vi "SetTimestampFormat.vi"(6 "time column mode (0: Empty)":T1, 8 "error in (no error)":errorcluster, 9 "absolulte time (T)":bool=TRUE, 10 "timestamp format":string, 11 "Excel refnum":T2) -> (0 "error out":errorcluster, 3 "Excel refnum out":T2)   [LabVIEW 2017, in "NI_ExcelFile.lvlib"]
doc: "Sets the time column mode and the format for every time column ( not written by the user) in a .xlsx file. Time column is used to record the time when writing data.\n \n\nExcel refnum: Specifies a reference to the .xlsx file on which to perform the operation. Use the Create VI to create or open the refnum.\n\ntimestamp format: Specifies the format for the time column. For example: YYYY/MM/DD hh:mm:ss.\n\nabsolute time: Specifies whether you want to use absolute or relative time for the data in the .xlsx file. If the value is TRUE, the time in the .xlsx file starts from the current time. If the value is FALSE, the time starts from 1904/01/01 00:00:00. The default is TRUE.This control is not valid if the data type is DDT or waveform because these data types already contain time information. \n\ntime column mode: Specifies whether you want to add time columns to the .xlsx file. If the value is Empty, this VI does not add any time column to this file. If the value is One, this VI adds one time column as the first column in this file. If the value is OnePerCh, this VI adds a time column to every data column in this file. The default is Empty.\n\nerror in: describes error conditions that occur before this node runs. This input provides standard error in functionality.\n\nExcel refnum out: Returns a Microsoft Excel file reference to the .xlsx file on which you performed the operation.\n\nerror out: contains error information. This output provides standard error out functionality."
uses:
  <vilib>/express/express shared/NI_ExcelFile/NI_ExcelFile.lvlib
  <vilib>/express/express shared/NI_ExcelFile/Ctrls/ExcelRefnum.ctl
  <vilib>/express/express shared/NI_ExcelFile/Ctrls/MainData.ctl
  <vilib>/express/express shared/NI_ExcelFile/Ctrls/StreamMode.ctl
  <vilib>/express/express shared/NI_ExcelFile/Ctrls/TimeColumnMode.ctl
  <vilib>/express/express shared/NI_ExcelFile/Ctrls/FileAttribute.ctl
  <vilib>/express/express shared/NI_ExcelFile/Ctrls/Columns.ctl
  <vilib>/express/express shared/NI_ExcelFile/Ctrls/ColumnInfo.ctl
  <vilib>/express/express shared/NI_ExcelFile/Ctrls/DataType.ctl
  <vilib>/express/express shared/NI_ExcelFile/Ctrls/wd_recordInfo.ctl
  <vilib>/express/express shared/NI_ExcelFile/Ctrls/disk_TemplateFile.ctl
  <vilib>/express/express shared/NI_ExcelFile/Ctrls/meta_file.ctl
  <vilib>/express/express shared/NI_ExcelFile/Ctrls/meta_Block.ctl
  <vilib>/express/express shared/NI_ExcelFile/Ctrls/meta_BlockType.ctl
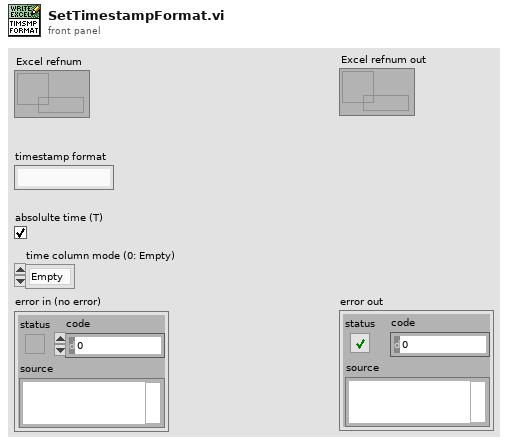
[diagram p1: front panel]
types:
  T1 = typedef "NI_ExcelFile.lvlib/TimeColumnMode.ctl" = enum16{"Empty", "OnePerCh", "One"}
  T2 = typedef "NI_ExcelFile.lvlib/ExcelRefnum.ctl" = refnum<data-value>
  T3 = typedef "NI_ExcelFile.lvlib/MainData.ctl" = cluster{"TargetFile":path, "StreamMode":T4, "Append?":bool, "ChunkSize":u64, "TimeColumnMode":T1, "TimestampFormat":string, "AbsoluteTime?":bool, "FileAttribute ":T5, "Column":T6, "FileRef":refnum<k1>, "MemoryRef":refnum<data-value>[], "RecordInfo":T9[], " ChannelPreviousInfo":u32[], "ChannelFirstRecord":u32[], "PredefinedFormattedValueLength":i64, "DiskTemplate":T10}
  T4 = typedef "NI_ExcelFile.lvlib/StreamMode.ctl" = enum16{"File", "Memory"}
  T5 = typedef "NI_ExcelFile.lvlib/FileAttribute.ctl" = cluster{"Creator":string, "Title":string, "SheetName":string}
  T6 = typedef "NI_ExcelFile.lvlib/Columns.ctl" = T7[]
  T7 = typedef "NI_ExcelFile.lvlib/ColumnInfo.ctl" = cluster{"Header":string, "Format":string, "DataType":T8, "Length":u64}
  T8 = typedef "NI_ExcelFile.lvlib/DataType.ctl" = enum16{"DDT", "WFM", "Array of STR", "Array of DBL", "Array of I8", "Array of I16", "Array of I32", "Array of I64", "Array of SGL", "Array of U8", "Array of U16", "Array of U32", "Array of U64", "Array of Time"}
  T9 = typedef "NI_ExcelFile.lvlib/wd_recordInfo.ctl" = cluster{"ChannelIndex":u32, "StartIndex":u64, "Length":u64, "Previous":i32, "Next":i32}
  T10 = typedef "NI_ExcelFile.lvlib/disk_TemplateFile.ctl" = cluster{"XMLRef":refnum<file>[], "ZipPath":path, "MetaFile":T11, "TempFolder":path}
  T11 = typedef "NI_ExcelFile.lvlib/meta_file.ctl" = cluster{"Ref":refnum<file>, "NextRow":i32, "NextPosition":i64, "Block":T12[]}
  T12 = typedef "NI_ExcelFile.lvlib/meta_Block.ctl" = cluster{"Version":u16, "Type":T13, "Length":i32, "Data":string}
  T13 = typedef "NI_ExcelFile.lvlib/meta_BlockType.ctl" = enum16{"NITag", "File", "Column"}
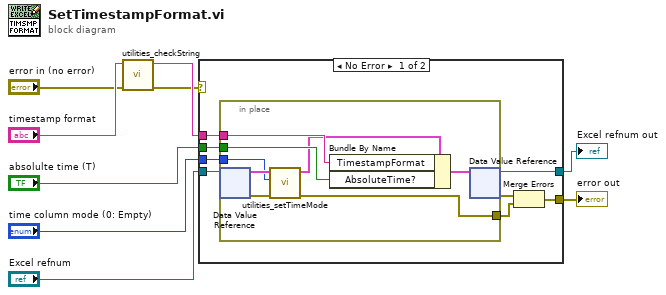
[diagram p0: block diagram]
diagram:
  n1 = call <vilib>:"utilities_checkString.vi"("error in (no error)"="error in (no error)", "String"="timestamp format") -> ("error out"=w1:errorcluster, "String out"=w3:string)  [unwired: 8 in]
  n2 = case shown="No Error" w1 {
    selector: w1 -> [_ w27]
    tunnel: [w12 w27] -> w9
    tunnel: w3 -> [w10 _]
    tunnel: "Excel refnum" -> [w17 w26]
    tunnel: [w16 w26] -> w7
    tunnel: "absolulte time (T)" -> [w15 _]
    tunnel: "time column mode (0: Empty)" -> [w11 _]
    frame No Error {
      n3 = in-place {
        in-place-border: w10 -> [w25]
        in-place-border: w15 -> [w24]
        in-place-border: [w19] -> w13
        in-place-border: w11 -> [w21]
        n4 = in-place-dvr #1(w17) -> (w23:T3, w20:errorcluster)
        n5 = call <vilib>:"utilities_setTimeMode.vi"("error in (no error)"=w20, "time column mode (0: Empty)"=w21, "data value"=w23) -> ("error out"=w19:errorcluster, "data value out"=w22:T3)  [unwired: 7 in]
        n6 = Bundle By Name(cluster=w22, "TimestampFormat"=w25, "AbsoluteTime?"=w24) -> (w18:T3)
        n7 = in-place-dvr #1(w18) -> (w16:T2, w14:errorcluster)
      }
      n8 = Merge Errors(w14, w13) -> (w12:errorcluster)
    }
    frame Error {
    }
  }
  "Excel refnum out" <- w7
  "error out" <- w9
